vi "Close Instrument Sessions.vi"(0 "SG Path Group in":refnum<class "SG 18GHz Path Group.lvclass">, 11 "error in (no error)":errorcluster) -> (4 "SG Path Group out":refnum<class "SG 18GHz Path Group.lvclass">, 15 "error out":errorcluster)   [LabVIEW 2023, in "RFFixtureCharact.RFPM.lvlib" / "SG 18GHz Path Group.lvclass"]
uses:
  SG 18GHz Path Group.lvclass
  Instruments/Power Meter/Power Meter Factory/Power Meter Factory.lvclass
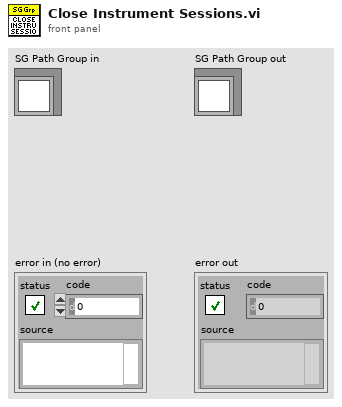
[diagram p1: front panel]
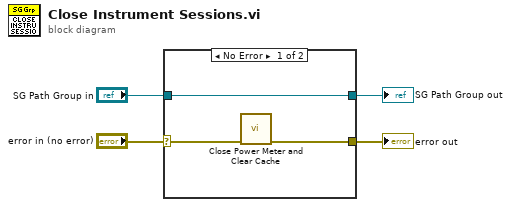
[diagram p0: block diagram]
diagram:
  n1 = case shown="No Error" "error in (no error)" {
    selector: "error in (no error)" -> [w5 w9]
    tunnel: [w7 w9] -> w4
    tunnel: [w6 w8] -> w2
    tunnel: "SG Path Group in" -> [w6 w8]
    frame No Error {
      n2 = call "Close Power Meter and Clear Cache.vi"("error in (no error)"=w5) -> ("error out"=w7:errorcluster)  [unwired: 14 in]
    }
    frame Error {
    }
  }
  "error out" <- w4
  "SG Path Group out" <- w2
